vi "Log.CreateChannelList.vi"(8 "error in (no error)":errorcluster, 9 "Station.ID":string, 10 "Value":T2(ring), 11 "Workspace":T1) -> (0 "error out":errorcluster, 3 "Channel List":T3[](array[typedef]))   [LabVIEW 2015, in "Single Station Execution.lvlib"]
uses:
  Single Station Execution.lvlib
  <vilib>/NI Veristand/Execution/DataLogging/TDMS Channel Group.ctl
  <vilib>/NI Veristand/Execution/DataLogging/TDMS Property.ctl
  <vilib>/NI Veristand/Execution/DataLogging/TDMS Channel.ctl
  <vilib>/NI Veristand/Execution/DataLogging/Time Channel Options.ctl
  <vilib>/NI Veristand/Execution/Workspace/WorkspaceAPI.ctl
  NationalInstruments.VeriStand.ClientAPI
  <vilib>/NI Veristand/Execution/DataLogging/NI_VS Data Logging API.lvlib
  <vilib>/NI Veristand/Execution/Workspace/NI_VS Workspace ExecutionAPI.lvlib
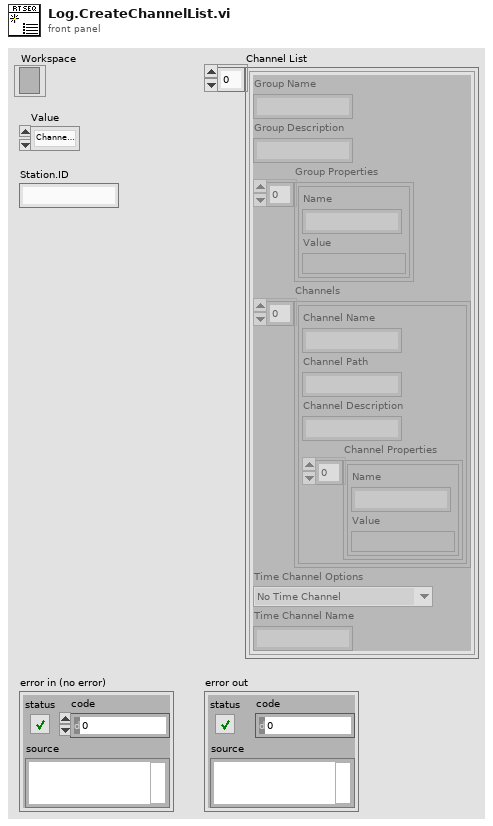
[diagram p1: front panel]
types:
  T1 = typedef "NI_VS Workspace ExecutionAPI.lvlib/WorkspaceAPI.ctl" = refnum<k24>
  T2 = enum16{"Channels (No System Channel)", "Aliases", "All"}
  T3 = typedef "NI_VS Data Logging API.lvlib/TDMS Channel Group.ctl" = cluster{"Group Name":string, "Group Description":string, "Group Properties":T4[], "Channels":T5[], "Time Channel Options":T6, "Time Channel Name":string}
  T4 = typedef "NI_VS Data Logging API.lvlib/TDMS Property.ctl" = cluster{"Name":string, "Value":variant}
  T5 = typedef "NI_VS Data Logging API.lvlib/TDMS Channel.ctl" = cluster{"Channel Name":string, "Channel Path":string, "Channel Description":string, "Channel Properties":T4[]}
  T6 = typedef "NI_VS Data Logging API.lvlib/Time Channel Options.ctl" = enum16{"No Time Channel", "Absolute Time", "System Time", "System Time - Microseconds", "Absolute Time as Double", "Relative To First Start Trigger", "Relative To Session Start"}
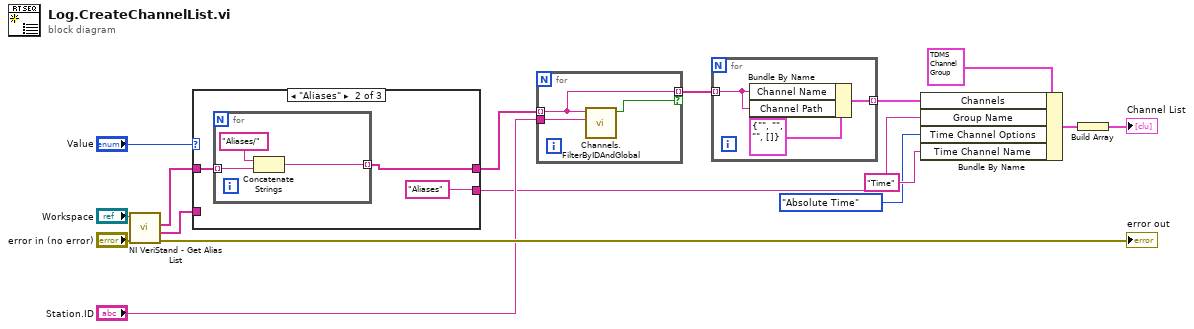
[diagram p0: block diagram]
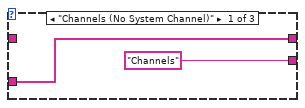
[diagram p2: hidden frame]
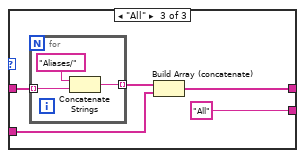
[diagram p3: hidden frame]
diagram:
  n1 = call <vilib>:"NI VeriStand - Get Alias List.vi"("error in (no error)"="error in (no error)", "WorkspaceManager in"="Workspace") -> ("error out"=→"error out":errorcluster, "Channels"=w5:string[], "Aliases"=w4:string[])  [unwired: 6 in, 1 out]
  n2 = case shown="\"Aliases\"" "Value" {
    tunnel: w4 -> [_ w21 w29]
    tunnel: [w18 w19 w27] -> w13
    tunnel: w5 -> [w18 _ w26]
    tunnel: ["Channels" "Aliases" "All"] -> w12
    frame "Channels (No System Channel)" {
    }
    frame "Aliases" {
      n3 = for {
        tunnel: w21 -> [w24] mode=indexing
        tunnel: [w22] -> w19 mode=indexing
        n4 = Concatenate Strings("Aliases/", w24) -> (w22:string)
      }
    }
    frame "All" {
      n5 = for {
        tunnel: w29 -> [w32] mode=indexing
        tunnel: [w30] -> w28 mode=indexing
        n6 = Concatenate Strings("Aliases/", w32) -> (w30:string)
      }
      n7 = Build Array (concatenate)(w28, w26) -> (w27:string[])
    }
  }
  n8 = for {
    tunnel: w13 -> [w35] mode=indexing
    tunnel: [w35] -> w14 mode=indexing if=w34
    tunnel: "Station.ID" -> [w33]
    n9 = call "Channels.FilterByIDAndGlobal.vi"("Station.ID"=w33, "Channel"=w35) -> ("Use?"=w34:bool)  [unwired: 9 in]
  }
  n10 = for {
    tunnel: w14 -> [w37] mode=indexing
    tunnel: [w36] -> w7 mode=indexing
    n11 = Bundle By Name(cluster=T5 {"Channel Name"="", "Channel Path"="", "Channel Description"="", "Channel Properties"=[]} ("TDMS Channel"), "Channel Name"=w37, "Channel Path"=w37) -> (w36:T5)
  }
  n12 = Bundle By Name(cluster=T3 {"Group Name"="", "Group Description"="", "Group Properties"=[], "Channels"=[], "Time Channel Options"=enum."No Time Channel", "Time Channel Name"=""} ("TDMS Channel Group"), "Channels"=w7, "Group Name"=w12, "Time Channel Options"=Time_Channel_Options."Absolute Time", "Time Channel Name"="Time") -> (w10:T3)
  n13 = Build Array(w10) -> (→"Channel List":T3[])
